vi "Pololu.Mgr - Set Device Config for Channel.vi"(7 "Device":T1, 10 "Channel":u8, 11 "Devices":T1[](array[typedef])) -> (2 "Index":i32, 3 "Devices Out":T1[](array[typedef]))   [LabVIEW 2018]
uses:
  SubVIs/Pololu.Device Config.ctl
  SubVIs/Pololu.Device Range Config.ctl
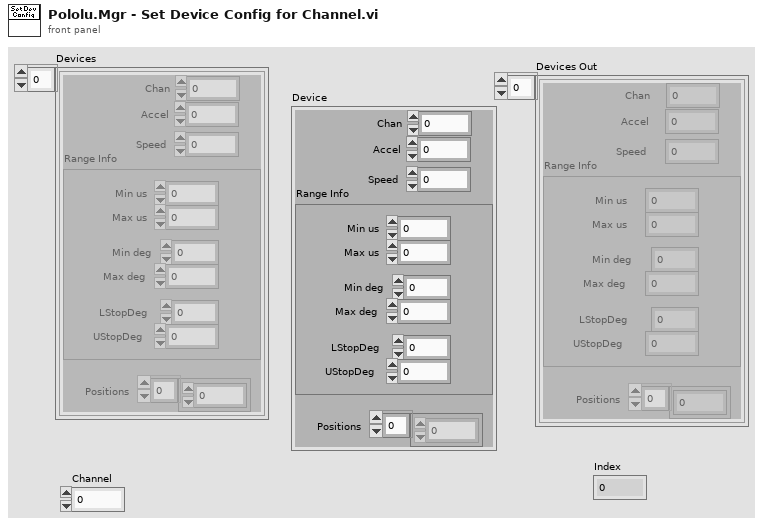
[diagram p1: front panel]
types:
  T1 = typedef "Pololu.Device Config.ctl" = cluster{"Chan":u8, "Accel":u16, "Speed":u16, "Positions":dbl[], "Range Info":T2}
  T2 = typedef "Pololu.Device Range Config.ctl" = cluster{"Min us":dbl, "Max us":dbl, "Min deg":dbl, "Max deg":dbl, "LStopDeg":dbl, "UStopDeg":dbl}
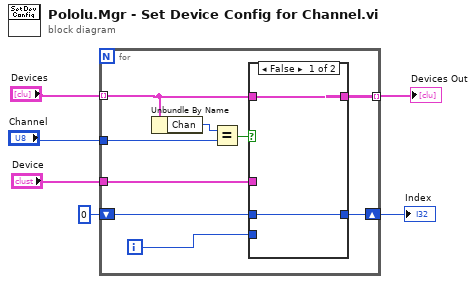
[diagram p0: block diagram]
diagram:
  n1 = for {
    tunnel: "Devices" -> [w10] mode=indexing
    tunnel: [w12] -> w3 mode=indexing
    tunnel: "Channel" -> [w14]
    tunnel: "Device" -> [w11]
    shift-right: [w9] -> w6
    shift-left: 0 -> [w7]
    i -> [w8]
    n2 = Unbundle By Name(w10) -> ("Chan"=w15:u8)
    n3 = Equal?(x=w15, y=w14) -> (x = y?=w13:bool)
    n4 = case shown="False" w13 {
      tunnel: [w17 w19] -> w12
      tunnel: w11 -> [_ w19]
      tunnel: w10 -> [w17 _]
      tunnel: [w16 w18] -> w9
      tunnel: w8 -> [_ w18]
      tunnel: w7 -> [w16 _]
      frame False {
      }
      frame True {
      }
    }
  }
  "Index" <- w6
  "Devices Out" <- w3
